vi "_InitInstrument.vi"(6 "GPIB as string":string, 7 "Channel":u8=255, 8 "error in (no error)":errorcluster, 9 "Name":string="null", 10 "VISA Resource Name":refnum<visa-resource-name>, 11 "Instrument in":refnum<class "Instrument.lvclass">) -> (0 "error out":errorcluster, 3 "Instrument out":refnum<class "Instrument.lvclass">)   [LabVIEW 2012, in "Instrument.lvclass"]
doc: "Superclass constructor: Protected access. Associate a name, and optionally a VISA Resource, with this Instrument. If Channel is specified, this constructor will append Channel to the Instrument's Name.\n\nCall this superclass constructor as the beginning of your subclass constructor. This will ensure you always operate on a valid Instrument. To ensure your subclass constructor produces objects of the correct type, ALWAYS connect your subclass constant to \"Instrument in\" on this superclass constructor."
uses:
  Instrument.lvclass
  Instrument.lvclass/Instrument.ctl
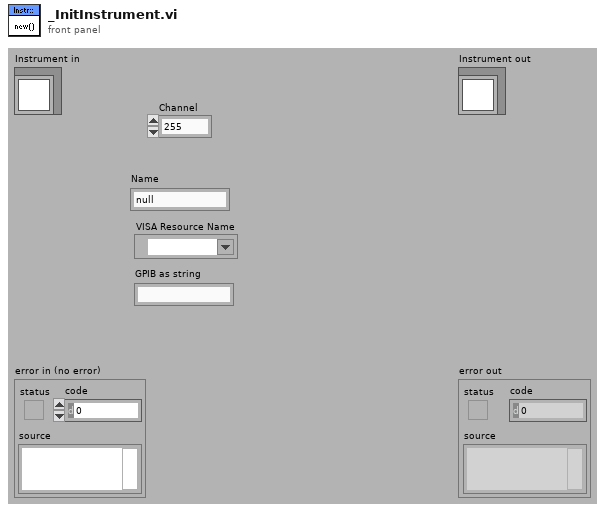
[diagram p1: front panel]
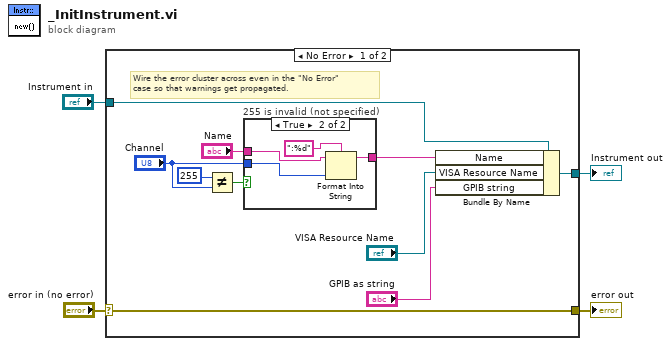
[diagram p0: block diagram]
diagram:
  n1 = case shown="No Error" "error in (no error)" {
    selector: "error in (no error)" -> [w13 w21]
    tunnel: [w13 w21] -> w3
    tunnel: [w12 w20] -> w1
    tunnel: "Instrument in" -> [w14 w20]
    frame No Error {
      # "Wire the error cluster across even in the \"No Error\"\ncase so that warnings get propagated."
      n2 = Not Equal?(x=255, y="Channel") -> (x != y?=w6:bool)
      n3 = case "255 is invalid (not specified)" shown="True" w6 {
        tunnel: "Channel" -> [_ w19]
        tunnel: "Name" -> [w15 w18]
        tunnel: [w15 w17] -> w10
        frame False {
        }
        frame True {
          n4 = Format Into String(format string=":%d", initial string=w18, w19) -> (resulting string=w17:string)  [unwired: 1 in, 1 out]
        }
      }
      n5 = Bundle By Name(cluster=w14, "Name"=w10, "VISA Resource Name"="VISA Resource Name", "GPIB string"="GPIB as string") -> (w12:refnum<class "Instrument.lvclass">)
    }
    frame Error {
    }
  }
  "error out" <- w3
  "Instrument out" <- w1
